vi "OceanOptics-v2.vi"(8 "Correct Electrical Dark":bool=TRUE, 10 "Average":i32=1, 11 "Integration Time (ms)":i32=100) -> (0 "XY Graph":T1(graph), 2 "Y":dbl[](array[numeric]), 3 "X":dbl[](array[numeric]))   [LabVIEW 2014]
doc: "André Romero - 2023\nandretec@ifsc.usp.br"
panel:
  out "Length":i32=3648
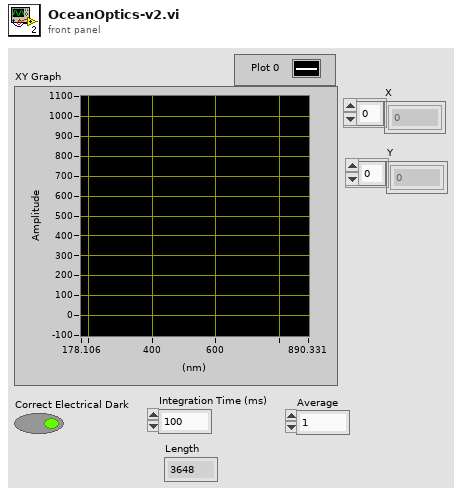
[diagram p1: front panel]
types:
  T1 = cluster{"WL Values":dbl[], "Spectrum Values":dbl[]}
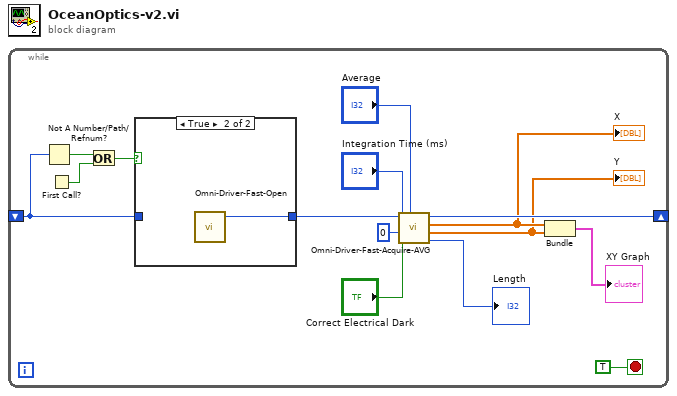
[diagram p0: block diagram]
diagram:
  n1 = while {
    shift-right: [w15] -> _
    shift-left: _ -> [w2]
    stop <- TRUE stop-if-true
    n2 = Not A Number/Path/Refnum?(number/path/refnum=w2) -> (NaN/Path/Refnum?=w6:bool)
    n3 = First Call?() -> (First Call?: T/F=w5:bool)
    n4 = Or(x=w6, y=w5) -> (x .or. y?=w3:bool)
    n5 = case shown="True" w3 {
      tunnel: [w16 w17] -> w4
      tunnel: w2 -> [w16 _]
      frame False {
      }
      frame True {
        n6 = call "Omni-Driver-Fast-Open.vi"() -> ("Wrapper Out"=w17:u32)  [unwired: 4 in, 1 out]
      }
    }
    n7 = call "Omni-Driver-Fast-Acquire-AVG.vi"("Average"="Average", "Correct Electrical Dark"="Correct Electrical Dark", "Spectrometer number"=0, "Integration Time (ms)"="Integration Time (ms)", "Wrapper"=w4) -> ("Length"=→"Length":i32, "Spectrum Values"=w10:dbl[], "WL Values"=w11:dbl[], "Wrapper Out"=w15:u32)
    "X" <- w11
    "Y" <- w10
    n8 = Bundle("WL Values"=w11, "Spectrum Values"=w10) -> (→"XY Graph":T1)  [unwired: 1 in]
  }
